vi "Configure Sweep.vi"(0 "VISA resource name":refnum<visa-resource-name>, 1 "Channel (1)":i32=1, 2 "Number of Measurement Points (201)":i32=201, 3 "Auto Sweep Time (F: Off)":bool, 5 "Sweep Time (0.001)":dbl=0.001 format="%^.3g", 9 "Delay Time (0.001)":dbl=0.001 format="%^.3g", 11 "error in (no error)":errorcluster, 12 "Sweep Mode (0: Stepped)":u16(ring) items=["Stepped", "Swept", "Fast Stepped Mode", "Fast Swept Mode", "Analog"], 13 "Sweep Type (0: Linear Sweep)":u16(ring) items=["Linear Sweep", "Logarithmic Sweep", "Segment Sweep", "Power Sweep", "DC Bias"], 14 "Configure Avoid Mode (F: Off)":bool) -> (4 "VISA resource name out":refnum<visa-resource-name>, 15 "error out":errorcluster)   [LabVIEW 2023, in "Agilent ENA Series.lvlib"]
doc: "Configures the sweep parameters."
uses:
  Agilent ENA Series.lvlib
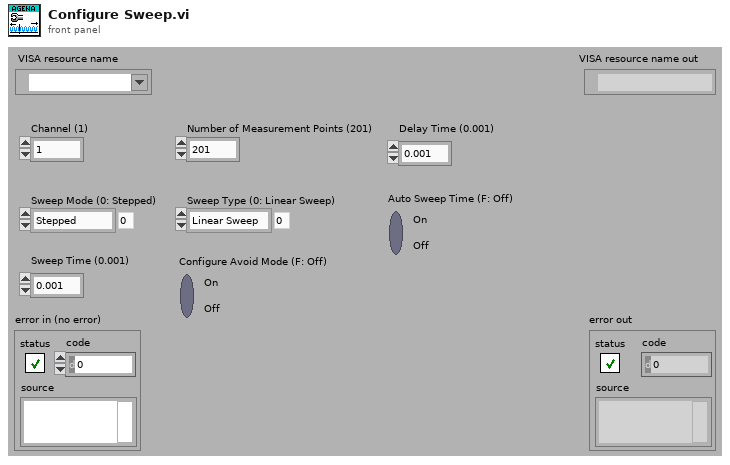
[diagram p1: front panel]
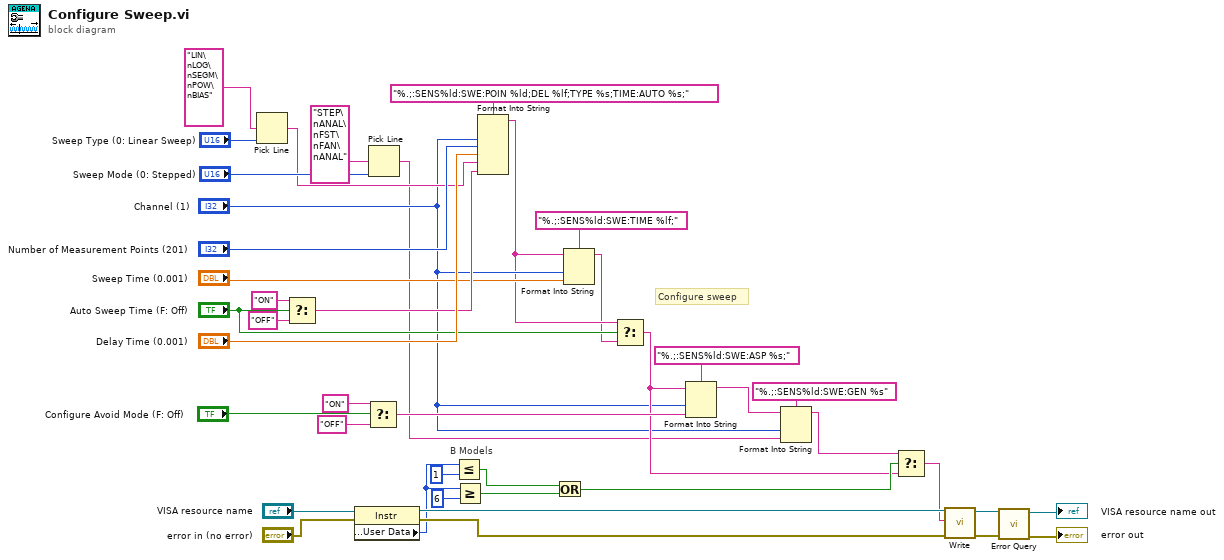
[diagram p0: block diagram]
diagram:
  # "Configure sweep"
  # "B Models"
  n1 = Pick Line(multi-line string="LIN\nLOG\nSEGM\nPOW\nBIAS", line index="Sweep Type (0: Linear Sweep)") -> (output string=w35:string)  [unwired: 1 in]
  n2 = Select(t="ON", s="Auto Sweep Time (F: Off)", f="OFF") -> (s? t:f=w32:string)
  n3 = property on="Property Node" class="Instr"(reference="VISA resource name", error in="error in (no error)") -> (reference out=w17:refnum<visa-resource-name>, error out=w16:errorcluster, "General Settings:User Data"=w6:u32)
  n4 = Select(t="ON", s="Configure Avoid Mode (F: Off)", f="OFF") -> (s? t:f=w21:string)
  n5 = Pick Line(multi-line string="STEP\nANAL\nFST\nFAN\nANAL", line index="Sweep Mode (0: Stepped)") -> (output string=w7:string)  [unwired: 1 in]
  n6 = Less Or Equal?(x=w6, y=u32 1) -> (x <= y?=w13:bool)
  n7 = Greater Or Equal?(x=w6, y=u32 6) -> (x >= y?=w14:bool)
  n8 = Format Into String(format string="%.;:SENS%ld:SWE:POIN %ld;DEL %lf;TYPE %s;TIME:AUTO %s;", "Channel (1)", "Number of Measurement Points (201)", "Delay Time (0.001)", w35, w32) -> (resulting string=w4:string)  [unwired: 2 in, 1 out]
  n9 = Or(x=w13, y=w14) -> (x .or. y?=w12:bool)
  n10 = Format Into String(format string="%.;:SENS%ld:SWE:TIME %lf;", initial string=w4, "Channel (1)", "Sweep Time (0.001)") -> (resulting string=w3:string)  [unwired: 1 in, 1 out]
  n11 = Select(t=w4, s="Auto Sweep Time (F: Off)", f=w3) -> (s? t:f=w11:string)
  n12 = Format Into String(format string="%.;:SENS%ld:SWE:ASP %s;", initial string=w11, "Channel (1)", w21) -> (resulting string=w10:string)  [unwired: 1 in, 1 out]
  n13 = Format Into String(format string="%.;:SENS%ld:SWE:GEN %s", initial string=w10, "Channel (1)", w7) -> (resulting string=w2:string)  [unwired: 1 in, 1 out]
  n14 = Select(t=w2, s=w12, f=w11) -> (s? t:f=w1:string)
  n15 = call "Write.vi"("error in (no error)"=w16, "String ()"=w1, "VISA resource name"=w17) -> ("error out"=w27:errorcluster, "VISA resource name out"=w28:refnum<visa-resource-name>)  [unwired: 6 in, 1 out]
  n16 = call "Error Query.vi"("error in (no error)"=w27, "VISA resource name"=w28) -> ("error out"=→"error out":errorcluster, "VISA resource name out"=→"VISA resource name out":refnum<visa-resource-name>)  [unwired: 6 in, 2 out]
